vi "DialogueNotesMarcoGonzalez.vi"() -> ()   [LabVIEW 2012]
panel:
  out "Color Box 2":u32(colorbox)
  out "Color Box":u32(colorbox)
  out "Boolean 2":bool
  out "Boolean 1":bool
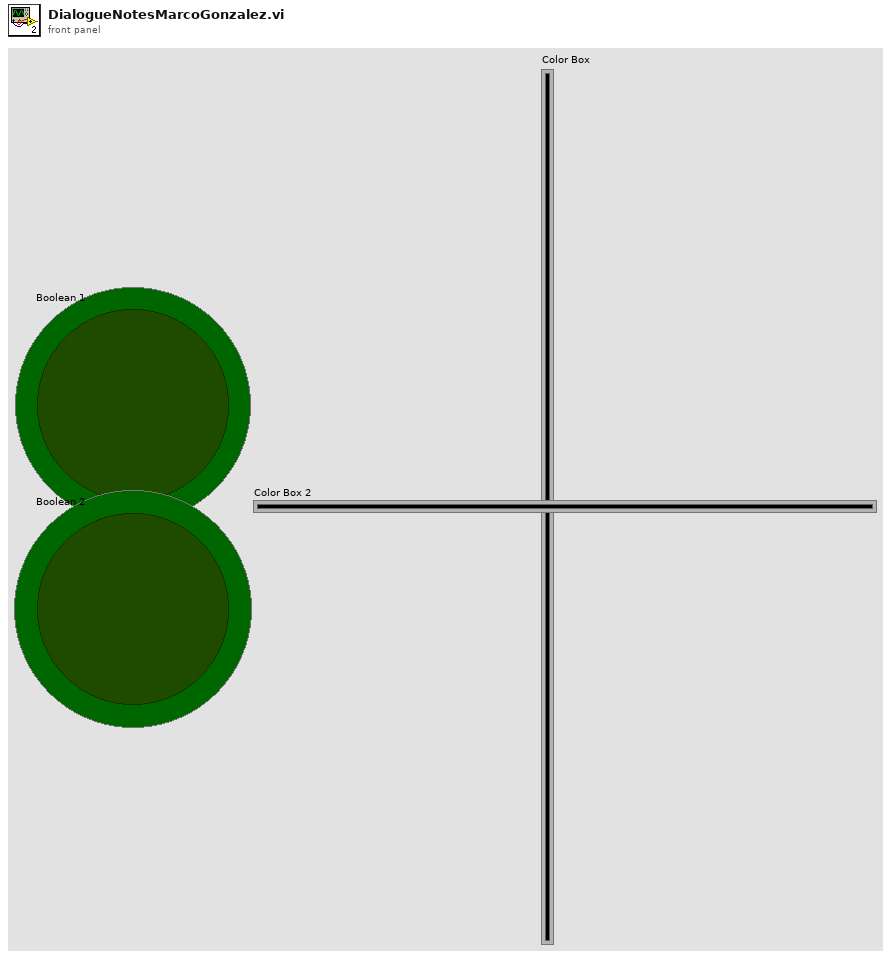
[diagram p1: front panel]
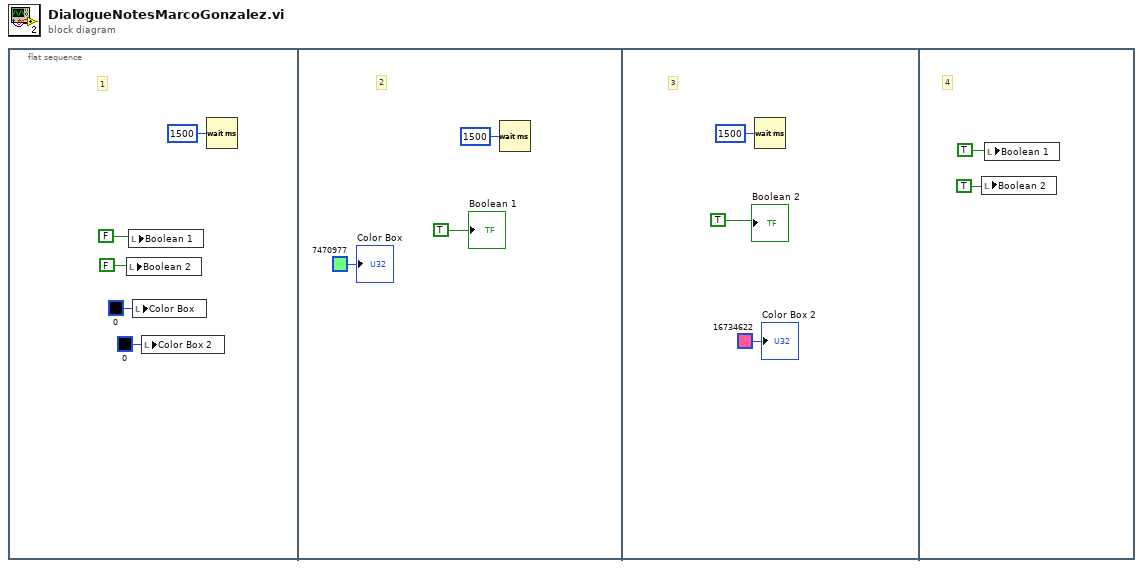
[diagram p0: block diagram]
diagram:
  n1 = flat-sequence {
    frame #0 {
      # "1"
      n2 = local write "Boolean 2"(FALSE) -> ()
      n3 = local write "Boolean 1"(FALSE) -> ()
      n4 = local write "Color Box"(u32 0 ("Color Box")) -> ()
      n5 = local write "Color Box 2"(u32 0 ("Color Box 2")) -> ()
      n6 = Wait (ms)(milliseconds to wait=u32 1500) -> ()  [unwired: 1 out]
    }
    frame #1 {
      # "2"
      n7 = Wait (ms)(milliseconds to wait=u32 1500) -> ()  [unwired: 1 out]
      "Boolean 1" <- TRUE
      "Color Box" <- u32 7470977 ("Color Box")
    }
    frame #2 {
      # "3"
      n8 = Wait (ms)(milliseconds to wait=u32 1500) -> ()  [unwired: 1 out]
      "Boolean 2" <- TRUE
      "Color Box 2" <- u32 16734622 ("Color Box 2")
    }
    frame #3 {
      # "4"
      n9 = local write "Boolean 2"(TRUE) -> ()
      n10 = local write "Boolean 1"(TRUE) -> ()
    }
  }
